vi "BME280_Create.vi"(0 "reference in":refnum<class "BME280.lvclass">, 3 "I2C Slave Address (0)":u8, 5 "error in (no error)":errorcluster) -> (14 "reference out":refnum<class "BME280.lvclass">, 19 "error out":errorcluster)   [LabVIEW 2014, in "BME280.lvclass"]
uses:
  BME280.lvclass
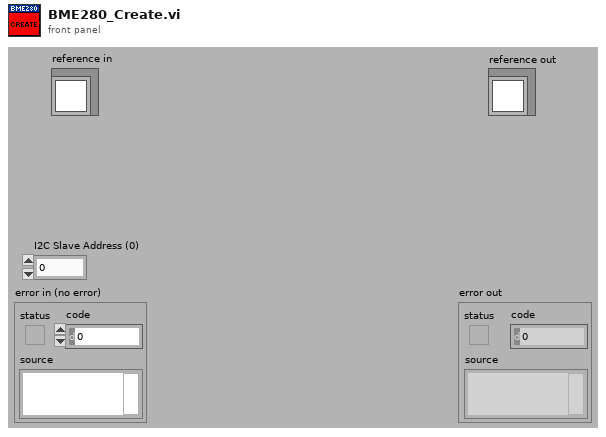
[diagram p1: front panel]
types:
  T1 = typedef "BME280.lvclass/ObjectAttributes.ctl" = cluster{"I2C Slave Address":u8, "TrimmingParameters":T2, "t_fine":i32}
  T2 = typedef "BME280.lvclass/TrimmingParameters.ctl" = cluster{"dig_T1":u16, "dig_T2":i16, "dig_T3":i16, "dig_P1":u16, "dig_P2":i16, "dig_P3":i16, "dig_P4":i16, "dig_P5":i16, "dig_P6":i16, "dig_P7":i16, "dig_P8":i16, "dig_P9":i16, "dig_H1":u8, "dig_H2":i16, "dig_H3":u8, "dig_H4":i16, "dig_H5":i16, "dig_H6":i8}
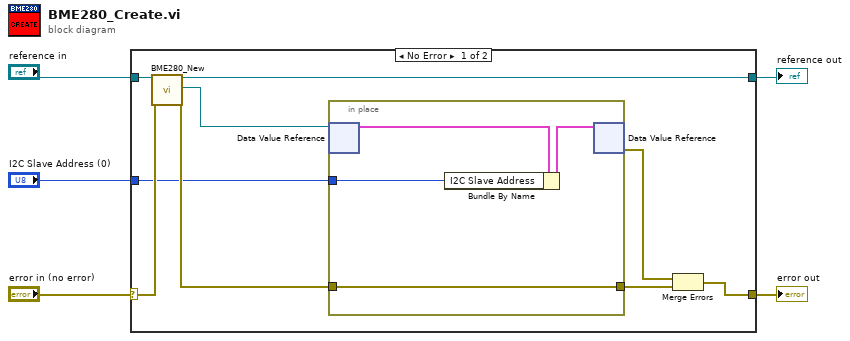
[diagram p0: block diagram]
diagram:
  n1 = case shown="No Error" "error in (no error)" {
    selector: "error in (no error)" -> [w13 w20]
    tunnel: [w10 w20] -> w4
    tunnel: "reference in" -> [w14 w19]
    tunnel: [w12 w19] -> w2
    tunnel: "I2C Slave Address (0)" -> [w6 _]
    frame No Error {
      n2 = call "BME280_New.vi"("reference in"=w14, "error in (no error)"=w13) -> ("reference out"=w12:refnum<class "BME280.lvclass">, "DVRRefOut"=w9:refnum<data-value>, "error out"=w8:errorcluster)  [unwired: 14 in, 1 out]
      n3 = in-place {
        in-place-border: w8 -> [w16]
        in-place-border: [w16] -> w7
        in-place-border: w6 -> [w15]
        n4 = in-place-dvr #1(w9) -> (w17:T1)  [unwired: 1 out]
        n5 = Bundle By Name(cluster=w17, "I2C Slave Address"=w15) -> (w18:T1)
        n6 = in-place-dvr #1(w18) -> (w11:errorcluster)  [unwired: 1 out]
      }
      n7 = Merge Errors(w11, w7) -> (w10:errorcluster)
    }
    frame Error {
    }
  }
  "error out" <- w4
  "reference out" <- w2
